vi "Test Suite Status on Fail.vi"(8 "error in (no error)":errorcluster, 11 "Test Suite Result Test In":refnum<class "Test Suite Result Test.lvclass">) -> (0 "error out":errorcluster, 3 "Test Suite Result Test Out":refnum<class "Test Suite Result Test.lvclass">)   [LabVIEW 2020, in "LUnit Tests.lvlib" / "Test Suite Result Test.lvclass"]
uses:
  Test Suite Result Test.lvclass
  C:/Program Files (x86)/National Instruments/LabVIEW 2020/vi.lib/Asteme/LUnit/Test Case.lvclass
  source/Examples/Basic Example/Failing Test Case/Failing Test Case.lvclass
  C:/Users/anton/Documents/GitHub/LUnit/source/Framework/Test Case/LUnit Test Case.lvclass
  source/Framework/Result Classes/Assertion Result/Public/TypeDefs/Status.ctl
  source/Framework/Result Classes/Test Suite Result/Test Suite Result.lvclass/Test Suite Result.ctl
  <vilib>/Asteme/LUnit/Test Case.lvclass/Test Case.ctl
  <vilib>/Asteme/LUnit/LUnit Assertion Result.lvclass/LUnit Assertion Result.ctl
  <vilib>/Asteme/LUnit/LUnit Test Case Result.lvclass/LUnit Test Case Result.ctl
  <vilib>/Asteme/LUnit/LUnit Method Result.lvclass/LUnit Method Result.ctl
  <vilib>/Asteme/LUnit/Palette/Fail.vi
  <vilib>/Asteme/LUnit/Palette/Pass.vi
  <vilib>/Asteme/LUnit/Set Assertion Type.vi
  <vilib>/Asteme/LUnit/Add test result.vi
  <vilib>/Asteme/LUnit/LUnit Write Passed.vi
  <vilib>/Asteme/LUnit/LUnit Write Message.vi
  <vilib>/Asteme/LUnit/LUnit Write Description.vi
  <vilib>/Asteme/LUnit/LUnit Write Assertion Type.vi
  <vilib>/Asteme/LUnit/LUnit Record Assertion Result.vi
  <vilib>/Asteme/LUnit/LUnit Aggregate Assertion Results.vi
  <vilib>/Asteme/LUnit/Assertion Result/LUnit Read Status.vi
  <vilib>/Asteme/LUnit/LUnit Read Message.vi
  <vilib>/Asteme/LUnit/LUnit Read Description.vi
  <vilib>/Asteme/LUnit/Method Result/LUnit Merge Status.vi
  <vilib>/Asteme/LUnit/LUnit Concatenate result strings.vi
  <vilib>/Asteme/LUnit/LUnit Assertion Result.lvclass
  source/Framework/Result Classes/Test Suite Result/Test Suite Result.lvclass
  <vilib>/Asteme/LUnit/Test Case.lvclass
  source/Framework/Result Classes/Assertion Result/Assertion Result.lvclass
  C:/Users/anton/Documents/GitHub/LUnit/source/Examples/Basic Example/Failing Test Case/Failing Test Case.lvclass
  C:/Users/anton/Documents/GitHub/LUnit/tests/Framework Test/Test Suite Result/Test Suite Result Test.lvclass
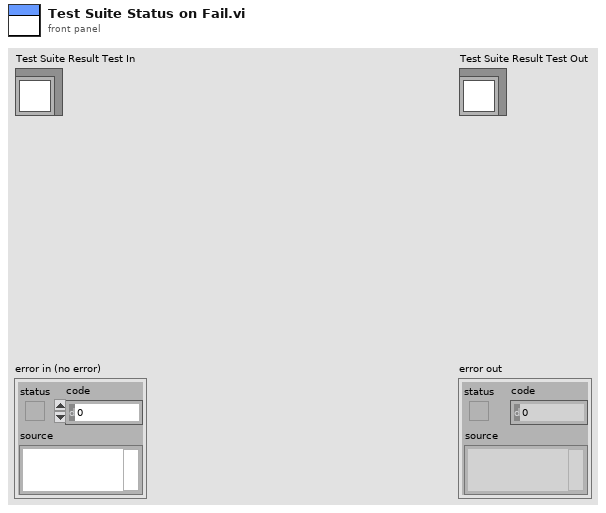
[diagram p1: front panel]
types:
  T1 = typedef "Assertion Result.lvclass/Status.ctl" = enum16{"Pass", "Fail", "Error", "Skipped", "Setup Error", "Broken", "Teardown Error"}
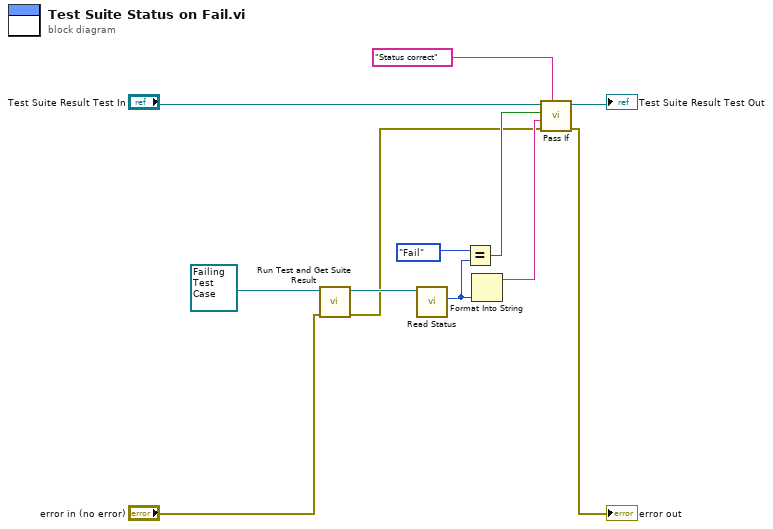
[diagram p0: block diagram]
diagram:
  n1 = call "Run Test and Get Suite Result.vi"("error in (no error)"="error in (no error)", "Test Test Case in"=refnum<class "Failing Test Case.lvclass"> refnum ("Failing Test Case.lvclass")) -> ("error out"=w1:errorcluster, "Test Suite Result out"=w4:refnum<class "Test Suite Result.lvclass">)  [unwired: 8 in]
  n2 = call "Read Status.vi"("Test Suite Result In"=w4) -> ("Status"=w6:T1)  [unwired: 9 in, 1 out]
  n3 = Equal?(x=Status."Fail" ("Status"), y=w6) -> (x = y?=w7:bool)
  n4 = Format Into String(w6) -> (resulting string=w5:string)  [unwired: 3 in, 1 out]
  n5 = call <vilib>:"Pass If.vi"("Description"="Status correct", "error in (no error)"=w1, "Message"=w5, "Pass?"=w7, "LUnit Test Case In"="Test Suite Result Test In") -> ("error out"=→"error out":errorcluster, "LUnit Test Case Out"=→"Test Suite Result Test Out":refnum<class "Test Suite Result Test.lvclass">)  [unwired: 5 in]
